vi "Personalities Directory.vi"(3 "Remote?":bool) -> (1 "appended path":path)   [LabVIEW 2019, in "Personalities Tool.lvlib"]
doc: "This VI returns the file directory where the personalities are stored."
uses:
  Personalities Tool.lvlib
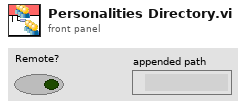
[diagram p1: front panel]
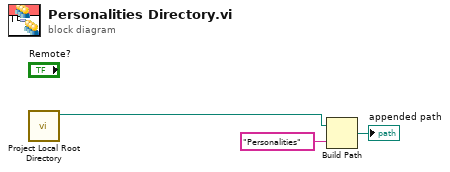
[diagram p0: block diagram]
diagram:
  n1 = call "Project Local Root Directory.vi"() -> ("Code root's folder"=w1:path)  [unwired: 11 in]
  n2 = Build Path(base path=w1, name or relative path="Personalities") -> (appended path=→"appended path":path)
